vi "Event handler-Back to origin.vi"   [LabVIEW 2020]
uses:
  Global Variables/gl_UI Ctrl Refs.vi
types:
  T1 = typedef "UI ctrl refs cluster.ctl" = cluster{"Top level VI path":path, "Top level VI ref":refnum<vi>, "User menu ref":refnum<k9>, "Sub Panel control":refnum<vi>, "Imaging Param Tab":refnum<vi>, "Occurrence-Start drivers":refnum<k4>, "Occurrence-Speed logging initialised":refnum<k4>, "Occurrence-XYZ stage initialised":refnum<k4>, "Exit button":refnum<vi>, "Status ind":refnum<vi>, "Set as origin":refnum<vi>, "Speed Logging":refnum<vi>, "Time Lapse":refnum<vi>, "Live Imaging":refnum<vi>, "AOL Z Stack":refnum<vi>, "Motor Z Stack":refnum<vi>, "Funct Acq button":refnum<vi>, "Hard Shutter":refnum<vi>, "Virtual Shutter":refnum<vi>, "Laser Power":refnum<vi>, "AOL Mode":refnum<vi>, "Frame Size":refnum<vi>, "Field of View":refnum<vi>, "Dwell Time":refnum<vi>, "Zoom":refnum<vi>, "AOL Z":refnum<vi>, "Objective":refnum<vi>, "Axis":refnum<vi>, "Paths & Names":refnum<vi>, "Experiment folder path (ind.)":refnum<vi>, "Last State (Ind.)":refnum<vi>, "Averages":refnum<vi>, "Angle (degrees)":refnum<vi>, "X centre":refnum<vi>, "Y centre":refnum<vi>, "Plane Mode":refnum<vi>, "# Planes":refnum<vi>, "Z Start":refnum<vi>, "Z Stop":refnum<vi>, "Z Step":refnum<vi>, "PMT 1":refnum<vi>, "PMT 2":refnum<vi>, "Stage XYZ Position":refnum<vi>, "Pockels@Z Start":refnum<vi>, "Pockels@Z Stop":refnum<vi>, "Obtain Z Start":refnum<vi>, "Obtain Z Stop":refnum<vi>, "Live stim.trig.period":refnum<vi>, "Live stim.trig.enable":refnum<vi>, "Movement Correction":refnum<vi>, "Load Reference Image":refnum<vi>, "XY Stage Move":refnum<vi>, "MovCor Cluster":refnum<vi>, "RefDAQParam":refnum<vi>, "Funct. Acq. Pockels Modulation":refnum<vi>, "Ref Laser Power":refnum<vi>, "Enable Video Recording":refnum<vi>, "Video Record-Live Imaging":refnum<vi>, "Video Record-Funct acq":refnum<vi>, "Reference Source":refnum<vi>, "AOL Z-stack Chirps Ready (ind)":refnum<vi>, "Target time between mov.cor. ref triggers (ms)":refnum<vi>, "Funct. Acq. Ref frame save":refnum<vi>, "Tracking button":refnum<vi>, "Show ref plots window":refnum<vi>, "Center freq ind (nm)":refnum<vi>, "Pickup mode (ind)":refnum<vi>, "Logging queue (ind)":refnum<vi>, "Back aperture power (ind.)":refnum<vi>, "Power after objective (ind.)":refnum<vi>, "Switch user":refnum<vi>, "Ls1 Conn. Status":refnum<vi>, "Ls1Tuning Status":refnum<vi>, "Ls1 Faults":refnum<vi>, "Ls1 Connection":refnum<vi>, "Ls1 Mode":refnum<vi>, "Ls1 POWER [mW]":refnum<vi>, "Ls1Shutter":refnum<vi>, "Ls1 Wavelength":refnum<vi>, "Ls1 Note":refnum<vi>, "Ls1 Confirm Wav":refnum<vi>, "Ls1 PreChrp Prism1":refnum<vi>, "Ls1 PreChrp Prism2":refnum<vi>, "Ls1 wav top Ind":refnum<vi>, "Ls1 power top Ind":refnum<vi>, "Ls1 Pump peak Hold":refnum<vi>, "Ls1 Status Ind":refnum<vi>, "Ls1 wav cancel":refnum<vi>, "Experiment Type":refnum<vi>, "Biology Information":refnum<vi>, "Camera recording status":refnum<vi>}
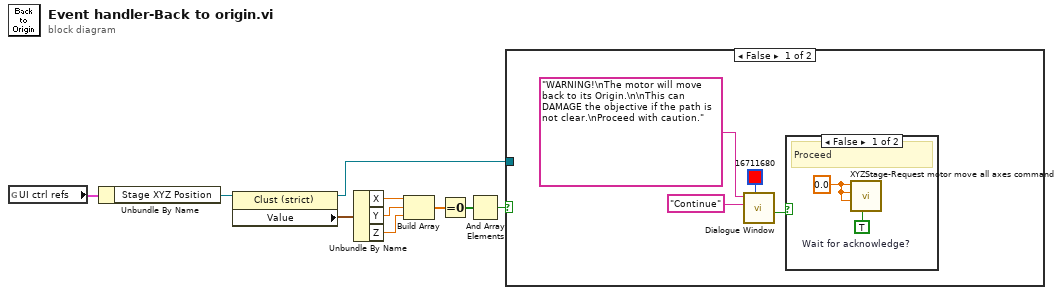
[diagram p0: block diagram]
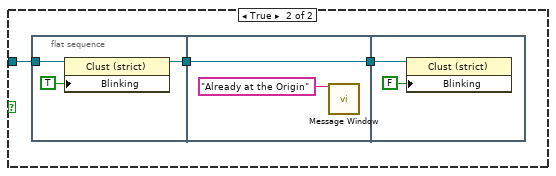
[diagram p3: hidden frame]
diagram:
  n1 = global read "gl_UI Ctrl Refs.vi" "UI ctrl refs"() -> (w10:T1)
  n2 = Unbundle By Name(w10) -> ("Stage XYZ Position"=w9:refnum<vi>)
  n3 = property class="Clust (strict)"(reference=w9) -> (reference out=w1:refnum<vi>, "Value"=w8:cluster{"X":sgl, "Y":sgl, "Z":sgl})  [unwired: 1 in, 1 out]
  n4 = Unbundle By Name(w8) -> ("X"=w7:sgl, "Y"=w6:sgl, "Z"=w5:sgl)
  n5 = Build Array(w7, w6, w5) -> (w4:sgl[])
  n6 = Equal To 0?(x=w4) -> (x = 0?=w3:bool[])
  n7 = And Array Elements(Boolean array=w3) -> (logical AND=w2:bool)
  n8 = case shown="False" w2 {
    tunnel: w1 -> [_ w19]
    frame False {
      n9 = call "Dialogue Window.vi"("Colour"=u32 16711680, "Caption-Right button (OK)"="Continue", "Message string"="WARNING!\nThe motor will move back to its Origin.\n\nThis can DAMAGE the objective if the path is not clear.\nProceed with caution.") -> ("Cancelled (Left button pressed)"=w13:bool)  [unwired: 6 in, 2 out]
      n10 = case shown="False" w13 {
        frame False {
          w15 = TRUE  # Wait for acknowledge?
          w16 = sgl 0.0 ("Motor X")
          # "Proceed"
          n11 = call "XYZStage-Request motor move all axes command.vi"("Wait for acknowledge?"=w15, "Motor Z"=w16, "Motor Y"=w16, "Motor X"=w16) -> ()  [unwired: 6 in, 2 out]
        }
        frame True {
          # "Cancelled"
        }
      }
    }
    frame True {
      n12 = flat-sequence {
        tunnel: w19 -> [w22]
        tunnel: [w20] -> w18
        tunnel: w18 -> [w24]
        tunnel: [w24] -> w17
        tunnel: w17 -> [w25]
        frame #0 {
          n13 = property class="Clust (strict)"(reference=w22, "Blinking"=TRUE) -> (reference out=w20:refnum<vi>)  [unwired: 1 in, 1 out]
        }
        frame #1 {
          n14 = call "Message Window.vi"("Message string"="Already at the Origin") -> ()  [unwired: 10 in, 1 out]
        }
        frame #2 {
          n15 = property class="Clust (strict)"(reference=w25, "Blinking"=FALSE) -> ()  [unwired: 1 in, 2 out]
        }
      }
    }
  }
